vi "Build Wheel Speed Sensor Section from XML.vi"(6 "Channels":refnum<k24>[](array[refnum]), 8 "error in (no error)":errorcluster, 9 "Card Position in":T1 {"Slot #" max=15}, 10 "Name in":string, 11 "Node Ptr in":u64) -> (0 "error out":errorcluster)   [LabVIEW 2014, in "SLSC configuration System Explorer.lvlib"]
uses:
  SLSC configuration System Explorer.lvlib
  Type Defs/Card Position.ctl
  Shared/SPI Utility/Slot #.ctl
  <vilib>/NI Veristand/Custom Device API/Custom Device Channel.ctl
  <vilib>/NI Veristand/Custom Device API/Custom Device Channel Type.ctl
  Shared/Constants.vi
  <vilib>/NI Veristand/Custom Device API/Set Item Property (U16).vi
  <vilib>/NI Veristand/Custom Device API/Custom Device API.lvlib
  Shared/SLSC configuration Shared.lvlib
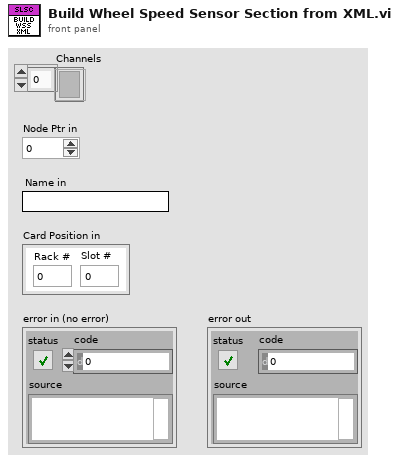
[diagram p1: front panel]
types:
  T1 = typedef "SLSC configuration Shared.lvlib/Card Position.ctl" = cluster{"Rack #":u8, "Slot #":T2}
  T2 = typedef "SLSC configuration Shared.lvlib/Slot #.ctl" = u8
  T3 = typedef "Custom Device API.lvlib/Custom Device Channel Type.ctl" = enum16{"Input", "Output"}
  T4 = typedef "Custom Device API.lvlib/Custom Device Channel.ctl" = cluster{"Type":T3, "Units":string, "Default Value":dbl, "Faultable":bool, "Scalable":bool}
  T5 = typedef "Custom Device API.lvlib/Custom Device Item Ref.ctl" = u64
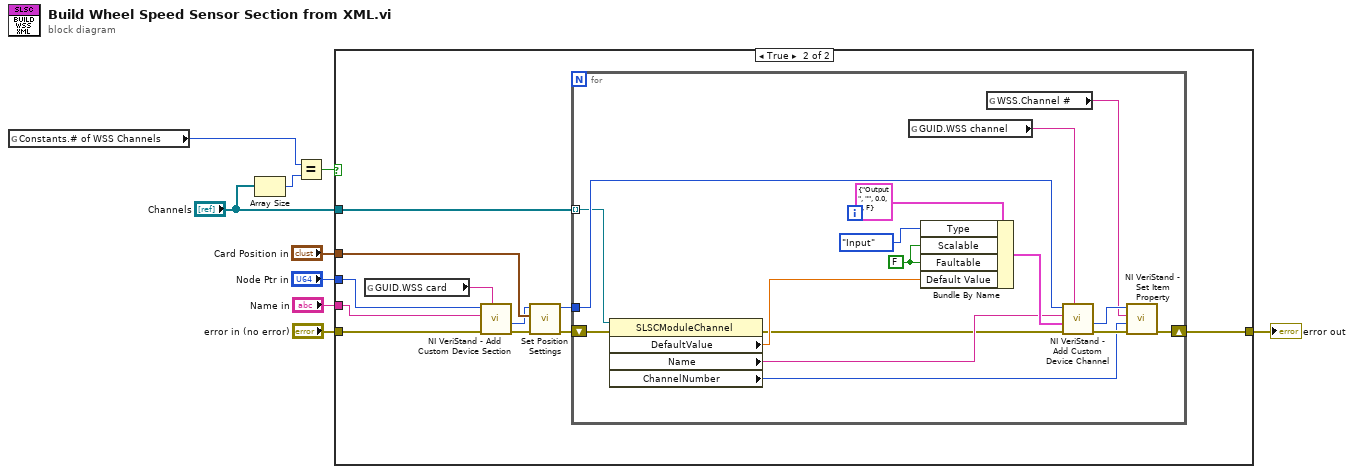
[diagram p0: block diagram]
diagram:
  n1 = global read "Constants.vi" "Constants.# of WSS Channels"() -> (w3:u8)
  n2 = Array Size(array="Channels") -> (size(s)=w4:i32)
  n3 = Equal?(x=w3, y=w4) -> (x = y?=w2:bool)
  n4 = case shown="True" w2 {
    tunnel: "error in (no error)" -> [w10 w21]
    tunnel: "Node Ptr in" -> [_ w20]
    tunnel: "Card Position in" -> [_ w17]
    tunnel: [w10 w11] -> w8
    tunnel: "Name in" -> [_ w13]
    tunnel: "Channels" -> [_ w12]
    frame False {
    }
    frame True {
      n5 = global read "Constants.vi" "GUID.WSS card"() -> (w19:string)
      n6 = call <vilib>:"NI VeriStand - Add Custom Device Section.vi"("GUID (Default Section)"=w19, "error in (no error)"=w21, "Section Name"=w13, "Parent Ref in"=w20) -> ("error out"=w18:errorcluster, "Section Ptr"=w16:T5)  [unwired: 4 in, 2 out]
      n7 = call "Set Position Settings.vi"("error in (no error)"=w18, "Card Position"=w17, "Item Ref in"=w16) -> ("error out"=w15:errorcluster, "Item Ref out"=w14:T5)  [unwired: 7 in]
      n8 = for {
        shift-right: [w28] -> w11
        shift-left: w15 -> [w27]
        tunnel: w14 -> [w31]
        tunnel: w12 -> [w26] mode=indexing
        w34 = FALSE ("Scalable")
        n9 = property class="SLSCModuleChannel"(reference=w26, error in=w27) -> (error out=w22:errorcluster, "DefaultValue"=w25:dbl, "Name"=w24:string, "ChannelNumber"=w23:u8)  [unwired: 1 out]
        n10 = global read "Constants.vi" "GUID.WSS channel"() -> (w33:string)
        n11 = Bundle By Name(cluster=T4 {"Type"=enum."Output", "Units"="", "Default Value"=0.0, "Faultable"=FALSE, "Scalable"=FALSE} ("Channel"), "Type"=Custom_Device_Channel_Type."Input", "Scalable"=w34, "Faultable"=w34, "Default Value"=w25) -> (w36:T4)
        n12 = global read "Constants.vi" "WSS.Channel #"() -> (w29:string)
        n13 = call <vilib>:"NI VeriStand - Add Custom Device Channel.vi"("GUID (Default Channel)"=w33, "error in (no error)"=w22, "Channel"=w36, "Channel Name"=w24, "Parent Ref in"=w31) -> ("error out"=w32:errorcluster, "Channel Ref"=w30:T5)  [unwired: 3 in, 2 out]
        n14 = call-poly <vilib>:"NI VeriStand - Set Item Property.vi"("error in (no error)"=w32, "Value"=w23, "Property Name"=w29, "Item Ref in"=w30) -> ("error out"=w28:errorcluster)  [unwired: 5 in, 2 out]
      }
    }
  }
  "error out" <- w8
